vi "save_asap_params.vi"() -> ()   [LabVIEW 2012]
uses:
  globals.vi
  <vilib>/Utility/xml.llb/Write to XML File(string).vi
panel:
  out "Input sample interval":dbl format="%#_6p"
  out "Output rate":dbl
  in  "Fs timebase":dbl=20000000.0 format="%#_6p"
  out "Half periods (sec)":dbl[](array[numeric])=[6.2e-05, 4.96e-05, 3.1e-05, 2.48e-05] format="%#_6p"
  in  "Desired output rate":dbl=1000.0 format="%#_6p"
  in  "Frequencies":string=" 59, 12, 13, 18, 16, 17, 19"
  in  "ASAP params file":path=path "c:/asap_params.xml"
  # "Input rate and carrier frequencies as multiples of the output rate.  Comma separated list, from Matlab script."
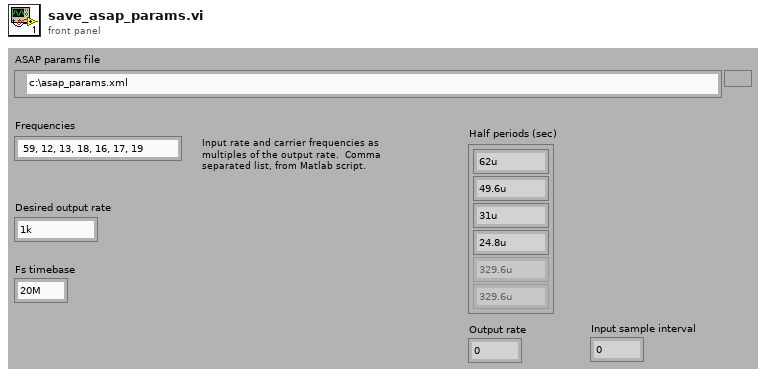
[diagram p1: front panel]
types:
  T1 = enum16{"ASAP/Trigger", "ASAP/Finder", "ASAP/Micron", "ASAP/Micron 2", "Micron 6DOF"}
  T2 = cluster{dbl, i32, "Num ASAP channels":i32, "Hardware version":enum16{"ASAP/Trigger", "ASAP/Finder", "ASAP/Micron", "ASAP/Micron 2", "Micron 6DOF"}, "Phase compensation (degrees)":dbl[][], dbl[], "Phase lags (degrees)":dbl[], "Gain calibration":sgl[][]}
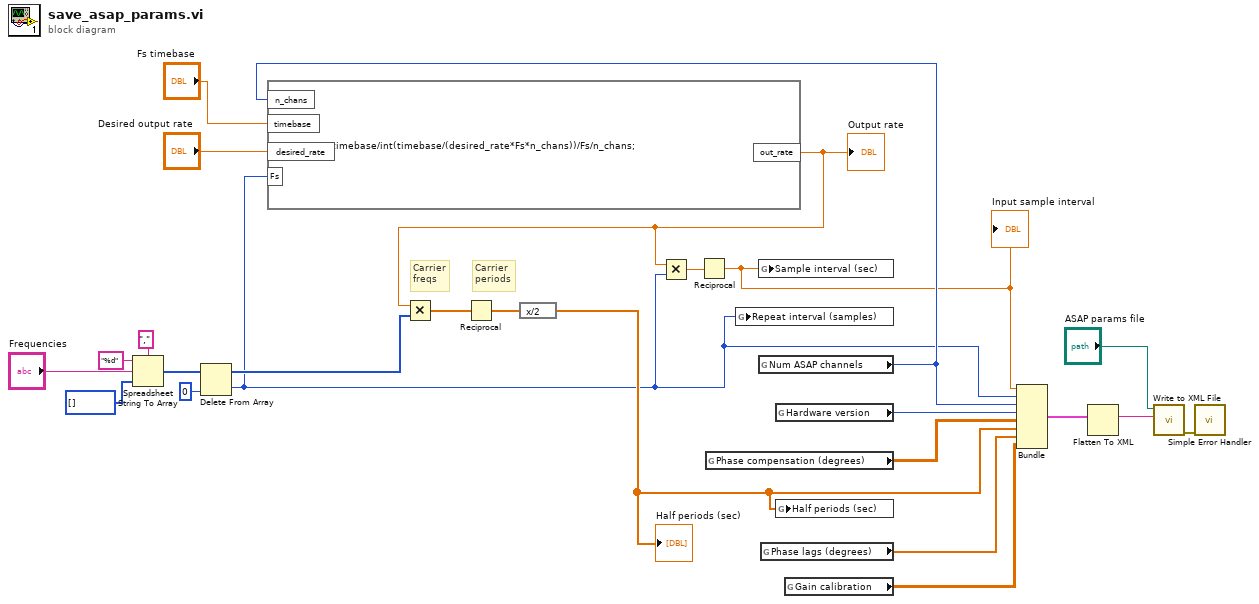
[diagram p0: block diagram]
diagram:
  # "Carrier\nperiods"
  # "Carrier\nfreqs"
  n1 = Spreadsheet String To Array(delimiter (Tab)=",", format string="%d", spreadsheet string="Frequencies", array type (2D Dbl)=i32[] []) -> (array=w15:i32[])
  n2 = Delete From Array(array=w15, index=0) -> (deleted portion=w5:i32, array with subset deleted=w13:i32[])  [unwired: 1 in]
  n3 = global read "globals.vi" "Phase compensation (degrees)"() -> (w24:dbl[][])
  n4 = global write "globals.vi" "Repeat interval (samples)"(w5) -> ()
  n5 = global read "globals.vi" "Num ASAP channels"() -> (w9:i32)
  n6 = formula code="out_rate = timebase/int(timebase/(desired_rate*Fs*n_chans))/Fs/n_chans;"("desired_rate"="Desired output rate", "Fs"=w5, "n_chans"=w9, "timebase"="Fs timebase") -> ("out_rate"=w4:dbl)
  "Output rate" <- w4
  n7 = Multiply(x=w4, y=w13) -> (x*y=w12:dbl[])
  n8 = Reciprocal(x=w12) -> (1/x=w11:dbl[])
  n9 = expression code="x/2"(w11) -> (w10:dbl[])
  "Half periods (sec)" <- w10
  n10 = Multiply(x=w4, y=w5) -> (x*y=w3:dbl)
  n11 = Reciprocal(x=w3) -> (1/x=w6:dbl)
  "Input sample interval" <- w6
  n12 = global write "globals.vi" "Sample interval (sec)"(w6) -> ()
  n13 = global read "globals.vi" "Phase lags (degrees)"() -> (w23:dbl[])
  n14 = global read "globals.vi" "Hardware version"() -> (w25:T1)
  n15 = global write "globals.vi" "Half periods (sec)"(w10) -> ()
  n16 = global read "globals.vi" "Gain calibration"() -> (w1:sgl[][])
  n17 = Bundle(w6, w5, "Num ASAP channels"=w9, "Hardware version"=w25, "Phase compensation (degrees)"=w24, w10, "Phase lags (degrees)"=w23, "Gain calibration"=w1) -> (w21:T2)  [unwired: 1 out]
  n18 = Flatten To XML(anything=w21) -> (xml string=w20:string)
  n19 = call-poly <vilib>:"Write to XML File.vi"("XML Input"=w20, "XML File Path"="ASAP params file") -> ("error out"=w22:errorcluster)  [unwired: 3 in, 6 out]
  n20 = call <vilib>:"Simple Error Handler.vi"("error in (no error)"=w22) -> ()  [unwired: 2 in, 7 out]
